vi "Compute Gated Decay (Tolerance).vi"(4 "Non Dirac IRF or non-0 lifetime":bool, 6 "tolerance":dbl, 8 "Error In":errorcluster, 9 "IRF Period":dbl, 10 "Gate & Decay Parameters Array":T1[](array[typedef]) {"A" format="%#_4g"; "s" format="%#_4g"; "sF" format="%#_4g"; "sR" format="%#_4g"; "t_i" format="%#_4g"; "t_0" format="%#_4g"; "tau" format="%#_4g"; "T" format="%#_4g"; "W" format="%#_4g"}, 11 "Time Points {t_i}":dbl[](array[numeric])) -> (0 "Error Out":errorcluster, 3 "{F(t_i)}":dbl[](array[numeric]))   [LabVIEW 2019]
uses:
  Gate & Decay Parameters.ctl
  Gate Type.ctl
  IRF Model.ctl
  Graphs/XY Graph/XY Plot Data.ctl
  Phasor_Abort Parallel Computation.vi
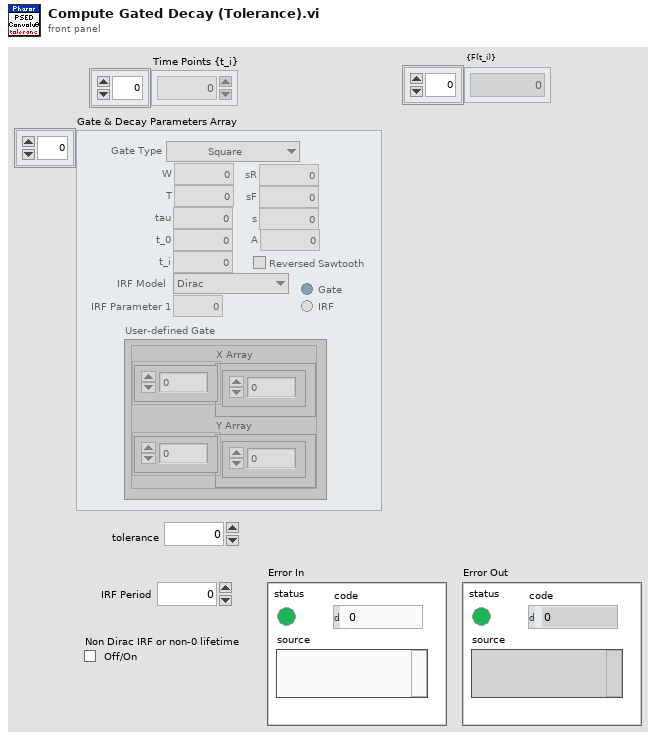
[diagram p1: front panel]
types:
  T1 = typedef "Gate & Decay Parameters.ctl" = cluster{"W":dbl, "T":dbl, "tau":dbl, "t_0":dbl, "Gate Type":T2, "t_i":dbl, "sR":dbl, "sF":dbl, "s":dbl, "Reversed Sawtooth":bool, "IRF Model":T3, "IRF Parameter 1":dbl, "User-defined Gate":T4, "Type of User-defined Function":enum32{"Gate", "IRF"}, "A":dbl}
  T2 = typedef "Gate Type.ctl" = enum16{"Square", "Finite Edge Square", "Finite Edge, Tilted Top Square", "Triangle", "Sawtooth", "User-defined"}
  T3 = typedef "IRF Model.ctl" = enum16{"Dirac", "Exponential"}
  T4 = typedef "XY Plot Data.ctl" = cluster{"X Array":dbl[], "Y Array":dbl[]}
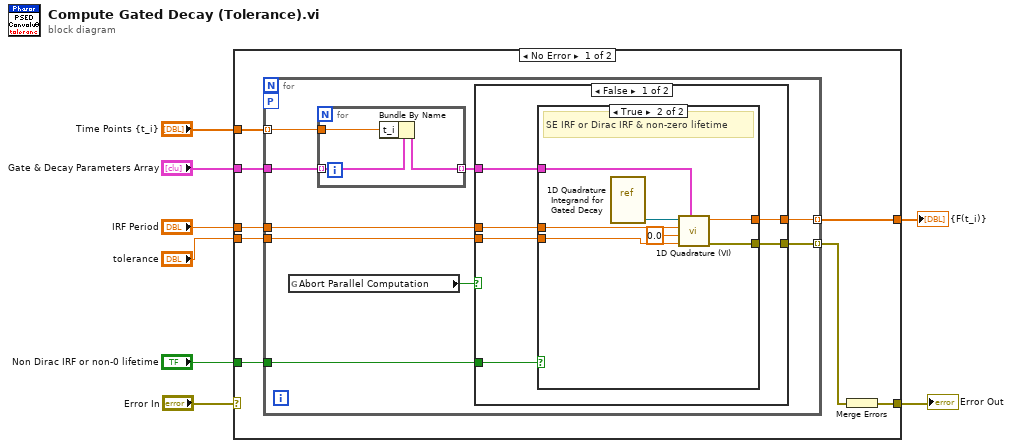
[diagram p0: block diagram]
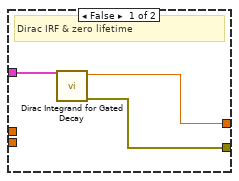
[diagram p2: hidden frame]
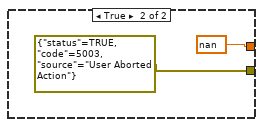
[diagram p3: hidden frame]
diagram:
  n1 = case shown="No Error" "Error In" {
    selector: "Error In" -> [_ w47]
    tunnel: "Non Dirac IRF or non-0 lifetime" -> [w16 _]
    tunnel: "IRF Period" -> [w15 _]
    tunnel: "tolerance" -> [w14 _]
    tunnel: [w13 _] -> w5
    tunnel: "Gate & Decay Parameters Array" -> [w12 _]
    tunnel: "Time Points {t_i}" -> [w11 _]
    tunnel: [w9 w47] -> w1
    frame No Error {
      n2 = for {
        tunnel: w11 -> [w21] mode=indexing
        tunnel: w12 -> [w20]
        tunnel: [w25] -> w13 mode=indexing
        workers-P: _ -> [_]
        tunnel: [w23] -> w10 mode=indexing
        tunnel: w14 -> [w24]
        tunnel: w15 -> [w22]
        tunnel: w16 -> [w18]
        n3 = global read "Phasor_Abort Parallel Computation.vi" "Abort Parallel Computation"() -> (w17:bool)
        n4 = for {
          tunnel: w21 -> [w28]
          tunnel: w20 -> [w27] mode=indexing
          tunnel: [w26] -> w19 mode=indexing
          n5 = Bundle By Name(cluster=w27, "t_i"=w28) -> (w26:T1)
        }
        n6 = case shown="False" w17 {
          tunnel: w19 -> [w34 _]
          tunnel: [w33 nan ("result")] -> w25
          tunnel: [w32 errorcluster {"status"=TRUE, "code"=5003, "source"="User Aborted Action"} ("error out")] -> w23
          tunnel: w24 -> [w31 _]
          tunnel: w22 -> [w30 _]
          tunnel: w18 -> [w29 _]
          frame False {
            n7 = case shown="True" w29 {
              tunnel: [w36 w44] -> w33
              tunnel: w34 -> [w37 w43]
              tunnel: [w35 w42] -> w32
              tunnel: w31 -> [_ w41]
              tunnel: w30 -> [_ w39]
              frame False {
                # "Dirac IRF & zero lifetime"
                n8 = call "Dirac Integrand for Gated Decay.vi"("data"=w37) -> ("Error Out"=w35:errorcluster, "F(X)"=w36:dbl)  [unwired: 9 in]
              }
              frame True {
                # "SE IRF or Dirac IRF & non-zero lifetime"
                n9 = vi-ref "1D Quadrature Integrand for Gated Decay.vi"() -> (w38:refnum<vi>)
                n10 = call "1D Quadrature (VI).vi"("data"=w43, "tolerance"=w41, "lower limit"=0.0, "upper limit"=w39, "integrand"=w38) -> ("Error Out"=w42:errorcluster, "result"=w44:dbl)  [unwired: 5 in]
              }
            }
          }
          frame True {
          }
        }
      }
      n11 = Merge Errors(w10) -> (w9:errorcluster)
    }
    frame Error {
    }
  }
  "{F(t_i)}" <- w5
  "Error Out" <- w1
